vi "Do.vi"(8 "error in (no error)":errorcluster, 10 "Actor in":refnum<class "Actor.lvclass">, 11 "Test Update Boolean Event Msg":refnum<class "Test Update Boolean Event Msg.lvclass">) -> (0 "error out":errorcluster, 2 "Actor out":refnum<class "Actor.lvclass">)   [LabVIEW 2016, in "Example Controller Actor.lvlib" / "Test Update Boolean Event Msg.lvclass"]
doc: "(<B>Filename</B>: Actor Framework.lvlib:Message.lvclass:Do.vi)\n\nDefines what a message does when it is received by an actor. Generally, a message instructs an actor to invoke one of its methods. By default, this method does nothing. A child class must override it to define behavior. Create a child class by using the Actor Framework Message Maker dialog box."
uses:
  Test Update Boolean Event Msg.lvclass
  C:/Project/Shared Libraries/Event Actors/Event Handlers/Event Generated Msg/Event Generated Msg.lvclass
  <vilib>/ActorFramework/Actor/Actor.lvclass
  Example Controller Actor.lvclass
  C:/Program Files (x86)/National Instruments/LabVIEW 2016/vi.lib/ActorFramework/Actor/Actor.lvclass
  Example Events/Boolean Event.lvclass
  Event Handlers/Event Generated Msg/Event Generated Msg.lvclass/Event Generated Msg.ctl
  Example Events/Boolean Event.lvclass/Boolean Event.ctl
  Event Handlers/Event Generated Msg/Event Generated Msg.lvclass
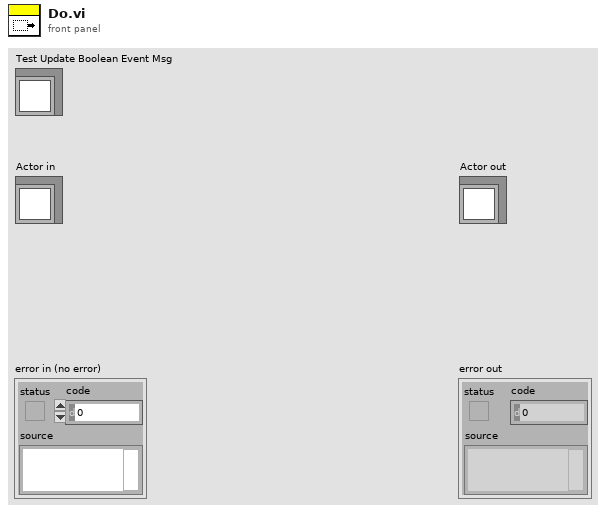
[diagram p1: front panel]
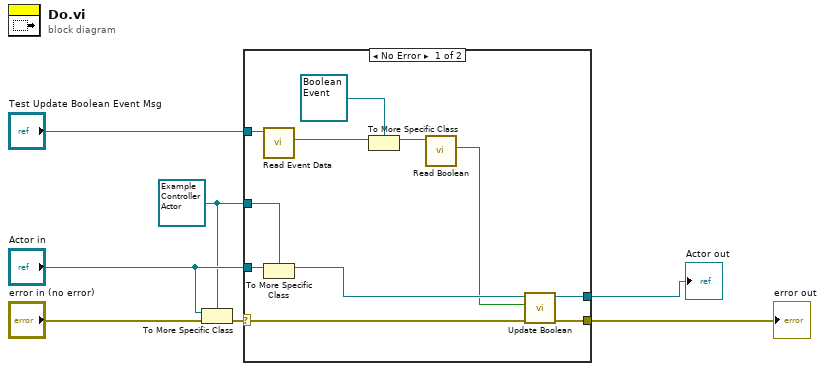
[diagram p0: block diagram]
diagram:
  w1 = refnum<class "Example Controller Actor.lvclass"> refnum ("Example Controller Actor.lvlib:Example Controller Actor.lvclass")
  n1 = To More Specific Class(target class=w1, reference="Actor in", error in="error in (no error)") -> (error out=w7:errorcluster)  [unwired: 1 out]
  n2 = case shown="No Error" w7 {
    selector: w7 -> [w16 w20]
    tunnel: [w18 w20] -> w3
    tunnel: [w17 w19] -> w2
    tunnel: "Actor in" -> [w15 w19]
    tunnel: w1 -> [w14 _]
    tunnel: "Test Update Boolean Event Msg" -> [w12 _]
    frame No Error {
      n3 = call "Read Event Data.vi"("Event Generated Msg"=w12) -> ("Event Data"=w11:refnum<class "Event.lvclass">)  [unwired: 10 in]
      n4 = To More Specific Class(target class=w14, reference=w15) -> (specific class reference=w13:refnum<class "Example Controller Actor.lvclass">)  [unwired: 1 in, 1 out]
      n5 = To More Specific Class(target class=refnum<class "Boolean Event.lvclass"> refnum ("Example Source.lvlib:Boolean Event.lvclass"), reference=w11) -> (specific class reference=w9:refnum<class "Boolean Event.lvclass">)  [unwired: 1 in, 1 out]
      n6 = call "Read Boolean.vi"("Double Array Event in"=w9) -> ("Boolean"=w8:bool)  [unwired: 9 in, 1 out]
      n7 = call "Update Boolean.vi"("error in (no error)"=w16, "Boolean"=w8, "Example Source in"=w13) -> ("error out"=w18:errorcluster, "Example Source out"=w17:refnum<class "Example Controller Actor.lvclass">)  [unwired: 7 in]
    }
    frame Error {
      # "If type check fails, pass the original object out again."
    }
  }
  "error out" <- w3
  "Actor out" <- w2
